vi "Set Tabs.vi"(9 "Enable/Disable Controls?":bool, 10 "Pages To Be Disabled":refnum<vi>[](array[refnum]), 11 "Pages To Be Enabled":refnum<vi>[](array[refnum])) -> ()   [LabVIEW 2014]
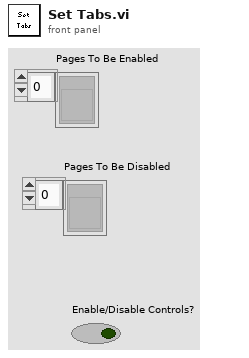
[diagram p1: front panel]
types:
  T1 = enum32{"Page Enabled", "Page Disabled", "Page Disabled & Grayed"}
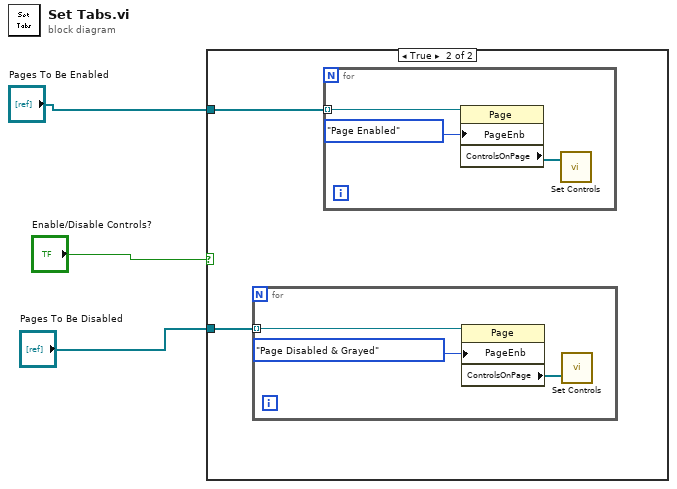
[diagram p0: block diagram]
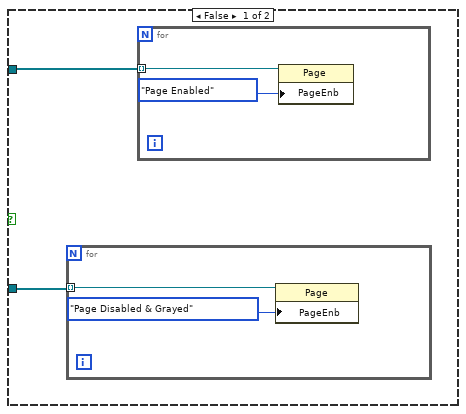
[diagram p2: hidden frame]
diagram:
  n1 = case shown="True" "Enable/Disable Controls?" {
    tunnel: "Pages To Be Disabled" -> [w4 w11]
    tunnel: "Pages To Be Enabled" -> [w5 w10]
    frame False {
      n2 = for {
        tunnel: w4 -> [w6] mode=indexing
        n3 = property class="Page"(reference=w6, "PageEnb"=T1."Page Disabled & Grayed" ("Page Enabled State")) -> ()  [unwired: 1 in, 2 out]
      }
      n4 = for {
        tunnel: w5 -> [w8] mode=indexing
        n5 = property class="Page"(reference=w8, "PageEnb"=T1."Page Enabled" ("Page Enabled State")) -> ()  [unwired: 1 in, 2 out]
      }
    }
    frame True {
      n6 = for {
        tunnel: w11 -> [w13] mode=indexing
        n7 = property class="Page"(reference=w13, "PageEnb"=T1."Page Disabled & Grayed" ("Page Enabled State")) -> ("ControlsOnPage"=w12:refnum<vi>[])  [unwired: 1 in, 2 out]
        n8 = call "Set Controls.vi"("Disabled Controls"=w12) -> ()  [unwired: 2 in]
      }
      n9 = for {
        tunnel: w10 -> [w16] mode=indexing
        n10 = property class="Page"(reference=w16, "PageEnb"=T1."Page Enabled" ("Page Enabled State")) -> ("ControlsOnPage"=w15:refnum<vi>[])  [unwired: 1 in, 2 out]
        n11 = call "Set Controls.vi"("Enabled Controls"=w15) -> ()  [unwired: 2 in]
      }
    }
  }
